vi "create_data_object.vi"(6 "Test":T1, 10 "packet size":i32, 11 "data size":i32) -> (3 "Test Data":T2)   [LabVIEW 2024, in "Tester.lvlib"]
uses:
  Tester.lvlib
  Tests/test_data--cluster.ctl
  Tests/packetized_data--cluster.ctl
  Tests/tests--enum.ctl
panel:
  out "encoded packets":string[](array[string])
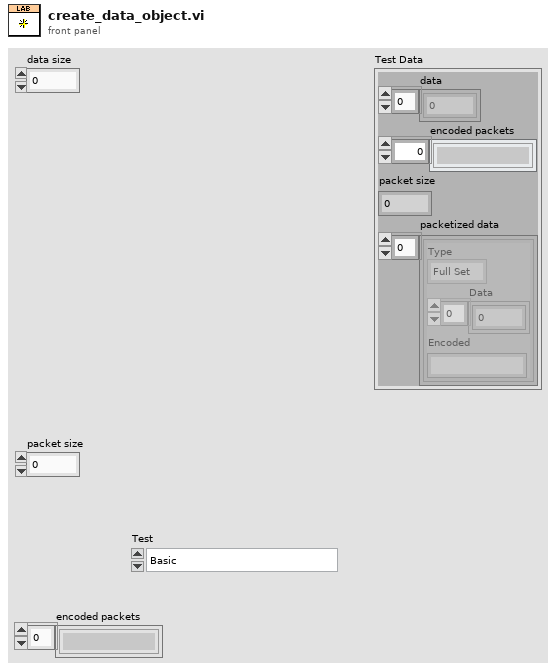
[diagram p1: front panel]
types:
  T1 = typedef "Tester.lvlib/tests--enum.ctl" = enum16{"Basic", "Pre-Allocated", "Packet-Type Case", "No IPE"}
  T2 = typedef "Tester.lvlib/test_data--cluster.ctl" = cluster{"data":dbl[], "encoded packets":string[], "packet size":i32, "packetized data":T3[]}
  T3 = typedef "Tester.lvlib/packetized_data--cluster.ctl" = cluster{"Type":enum16{"Full Set", "Last Set"}, "Data":dbl[], "Encoded":string}
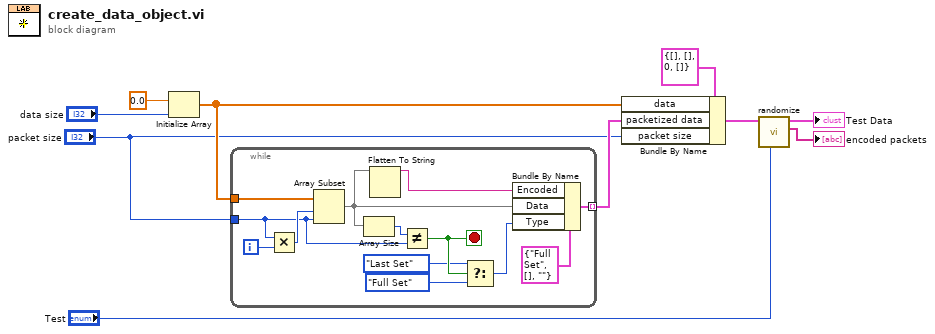
[diagram p0: block diagram]
diagram:
  n1 = Initialize Array(0.0, "data size") -> (w6:dbl[])
  n2 = while {
    tunnel: w6 -> [w23]
    tunnel: "packet size" -> [w19]
    tunnel: [w17] -> w5 mode=indexing
    i -> [w21]
    stop <- w15 stop-if-true
    n3 = Multiply(x=w19, y=w21) -> (x*y=w22:i32)
    n4 = Array Subset(array=w23, index=w22, length=w19) -> (w18:dbl[])
    n5 = Array Size(array=w18) -> (size(s)=w20:i32)
    n6 = Flatten To String(anything=w18) -> (data string=w16:string)  [unwired: 3 in, 2 out]
    n7 = Not Equal?(x=w20, y=w19) -> (x != y?=w15:bool)
    n8 = Select(t=enum16{"Full Set", "Last Set"}."Last Set" ("Type"), s=w15, f=enum16{"Full Set", "Last Set"}."Full Set" ("Type")) -> (s? t:f=w12:enum16{"Full Set", "Last Set"})
    n9 = Bundle By Name(cluster=T3 {"Type"=enum."Full Set", "Data"=[], "Encoded"=""} ("packetized data"), "Encoded"=w16, "Data"=w18, "Type"=w12) -> (w17:T3)
  }
  n10 = Bundle By Name(cluster=T2 {"data"=[], "encoded packets"=[], "packet size"=0, "packetized data"=[]} ("test data"), "data"=w6, "packetized data"=w5, "packet size"="packet size") -> (w8:T2)
  n11 = call "randomize.vi"("Test"="Test", "Test Data in"=w8) -> ("encoded packets"=→"encoded packets":string[], "Test Data out"=→"Test Data":T2)  [unwired: 8 in]
